vi "SS2 Live_Ready to Quit.vi"(8 "Error In":errorcluster, 9 "Flags":bool[](array[boolean]), 11 "SS2 Live Queue in":refnum<queue>) -> (0 "Error Out":errorcluster, 3 "Ready to Quit?":bool)   [LabVIEW 2019]
uses:
  SS2 Q [Element].ctl
  SS2 Q Event List.ctl
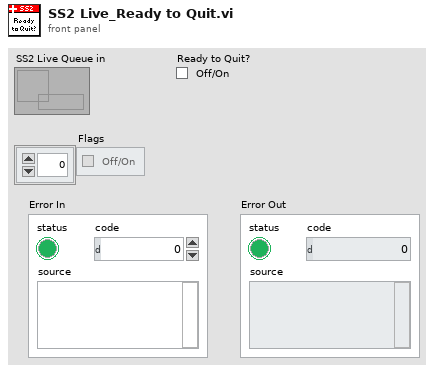
[diagram p1: front panel]
types:
  T1 = typedef "SS2 Q [Element].ctl" = cluster{"SS2 Q Event":T2, "Data":variant}
  T2 = typedef "SS2 Q Event List.ctl" = enum16{"---- UI ----", "Idle", "Initialization", "FPGA Status", "Quit", "---- DAQ ----", "Start Recording", "Start Live Acquisition", "Initialize Recording Mode", "Initialize FPGA (Live Mode)", "Get Image Set", "Get Single Image", "Update Image Display", "Stop Live Acquisition", "Stop Data Recording", "Stop Data Saving", "---- Image ----", "Copy Data to Clipboard", "Set Image Palette", "Save Displayed Image with Overlay", "Save Image Data as TIFF"}
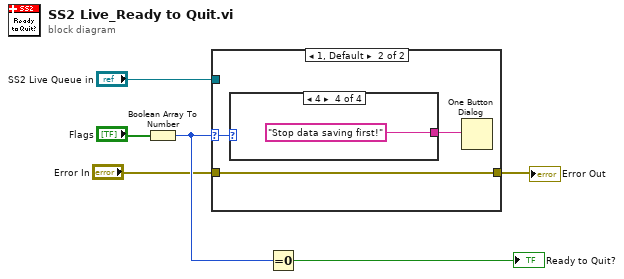
[diagram p0: block diagram]
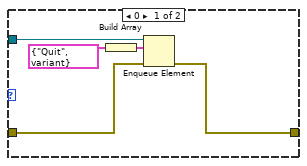
[diagram p2: hidden frame]
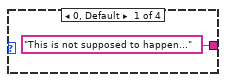
[diagram p3: hidden frame]
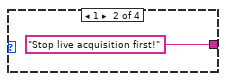
[diagram p4: hidden frame]
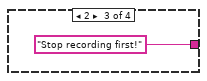
[diagram p5: hidden frame]
diagram:
  n1 = Boolean Array To Number(Boolean array="Flags") -> (number=w5:u32)
  n2 = case shown="1, Default" w5 {
    selector: w5 -> [_ w14]
    tunnel: "SS2 Live Queue in" -> [w11 _]
    tunnel: "Error In" -> [w8 w12]
    tunnel: [w7 w12] -> w1
    frame 0 {
      n3 = Build Array(T1 {"SS2 Q Event"=enum."Quit", "Data"=variant} ("element")) -> (w9:T1[])
      n4 = Enqueue Element(queue=w11, element=w9, error in (no error)=w8) -> (error out=w7:errorcluster)  [unwired: 1 in, 2 out]
    }
    frame 1, Default {
      n5 = case shown="4" w14 {
        tunnel: ["This is not supposed to happen..." ("message") "Stop live acquisition first!" ("message") "Stop recording first!" ("message") "Stop data saving first!" ("message")] -> w13
        frame 0, Default {
        }
        frame 1 {
        }
        frame 2 {
        }
        frame 4 {
        }
      }
      n6 = One Button Dialog(message=w13) -> ()  [unwired: 1 in, 1 out]
    }
  }
  "Error Out" <- w1
  n7 = Equal To 0?(x=w5) -> (x = 0?=→"Ready to Quit?":bool)
